vi "BM Configuration.vi"(8 "error in (no error)":errorcluster, 11 "Bus Monitor in":refnum<class "Bus Monitor.lvclass">) -> (0 "error out":errorcluster, 3 "Bus Monitor out":refnum<class "Bus Monitor.lvclass">)   [LabVIEW 2020, in "Unit Tests.lvlib" / "Bus Monitor.lvclass"]
uses:
  Bus Monitor.lvclass
  Bus Monitor.lvclass/Bus Monitor.ctl
  <vilib>/addons/_JKI Toolkits/Caraya/classes/Assert/Assert True.vi
  Dependencies/FPGA Interface/FPGA Interface.lvclass
  <vilib>/addons/_JKI Toolkits/Caraya/classes/Assert/Assert.lvclass
  <vilib>/addons/_JKI Toolkits/Caraya/classes/Test/Test.lvclass
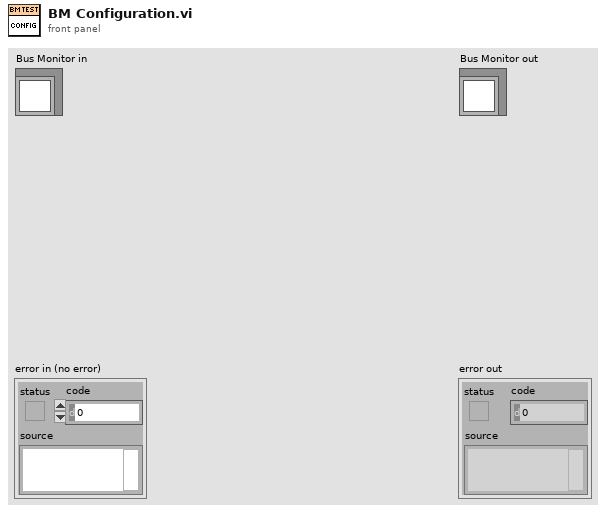
[diagram p1: front panel]
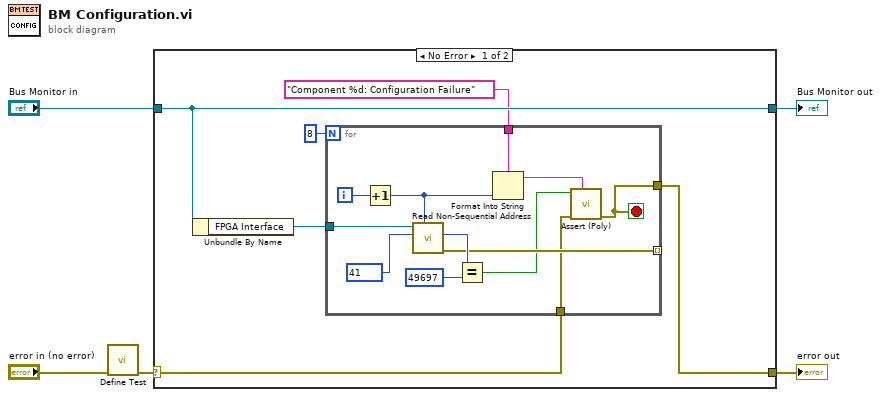
[diagram p0: block diagram]
diagram:
  n1 = call <vilib>:"Define Test.vi"("error in (no error)"="error in (no error)") -> ("error out"=w1:errorcluster)  [unwired: 9 in, 1 out]
  n2 = case shown="No Error" w1 {
    selector: w1 -> [w8 w25]
    tunnel: [w7 w25] -> w5
    tunnel: [w11 w24] -> w3
    tunnel: "Bus Monitor in" -> [w11 w24]
    frame No Error {
      n3 = Unbundle By Name(w11) -> ("FPGA Interface"=w10:refnum<class "FPGA Interface.lvclass">)
      n4 = for {
        N: 8 -> [_]
        tunnel: w10 -> [w23]
        tunnel: "Component %d: Configuration Failure" ("custom report message (\"\")") -> [w20]
        tunnel: w8 -> [w14]
        tunnel: [w15] -> w7
        tunnel: [w17] -> _ mode=indexing
        i -> [w22]
        stop <- w15 stop-if-true
        n5 = Increment(x=w22) -> (x+1=w19:i32)
        n6 = call-dynamic "Read Non-Sequential Address.vi"("Target IC (1-8)"=w19, "Address"=u16 41, "FPGA Interface in"=w23) -> ("error out"=w17:errorcluster, "Data"=w18:u16)  [unwired: 7 in]
        n7 = Equal?(x=w18, y=u16 49697) -> (x = y?=w13:bool)
        n8 = Format Into String(format string=w20, w19) -> (resulting string=w12:string)  [unwired: 2 in, 1 out]
        n9 = call-poly <vilib>:"Assert (Poly).vi"("Label"=w12, "error in (no error)"=w14, "True?"=w13) -> ("error out"=w15:errorcluster)  [unwired: 7 in, 1 out]
      }
    }
    frame Error {
    }
  }
  "error out" <- w5
  "Bus Monitor out" <- w3
